vi "Fetch N - Blob.vi"(8 "error in (no error)":errorcluster, 9 "n rows (-1:all)":i32=-1, 11 "SQLite3LV Cursor in":refnum<class "cursor.lvclass">) -> (0 "error out":errorcluster, 1 "rows finished?":bool, 2 "result":string[][](array[string]), 3 "SQLite3LV Cursor out":refnum<class "cursor.lvclass">)   [LabVIEW 2014, in "SQLite3LV.lvlib" / "cursor.lvclass"]
uses:
  cursor.lvclass
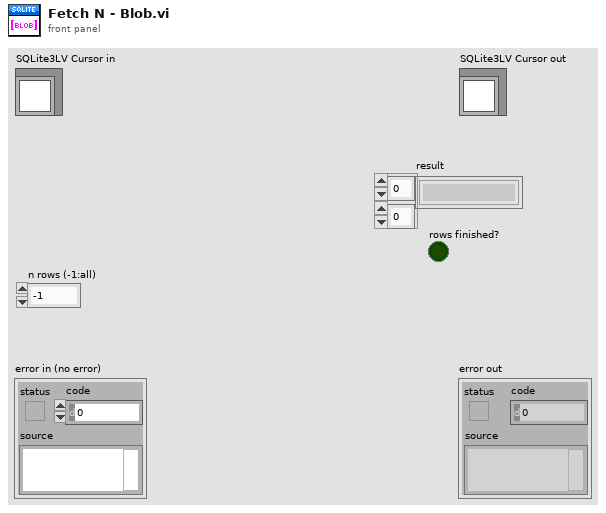
[diagram p1: front panel]
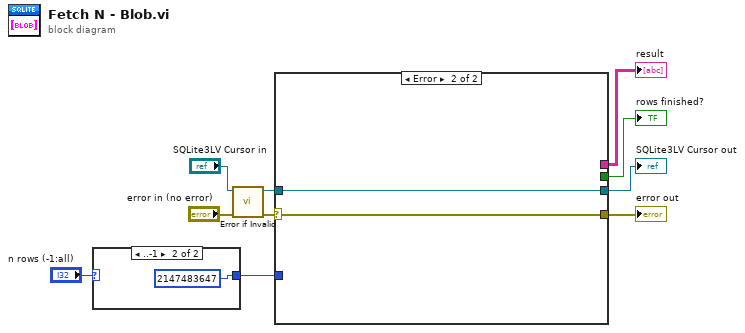
[diagram p0: block diagram]
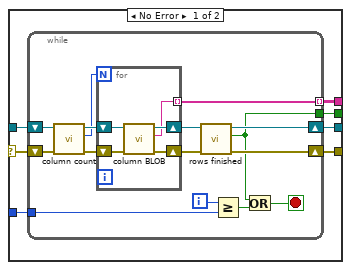
[diagram p3: hidden frame]
diagram:
  n1 = case shown="..-1" "n rows (-1:all)" {
    selector: "n rows (-1:all)" -> [w11 _]
    tunnel: [w11 2147483647 ("n rows (-1:all)")] -> w7
    frame Default {
    }
    frame ..-1 {
    }
  }
  n2 = call "Error if Invalid.vi"("error in (no error)"="error in (no error)", "SQLite3LV Cursor in"="SQLite3LV Cursor in") -> ("error out"=w2:errorcluster, "SQLite3LV Cursor out"=w3:refnum<class "cursor.lvclass">)  [unwired: 8 in]
  n3 = case shown="Error" w2 {
    selector: w2 -> [w18 w41]
    tunnel: [w15 w41] -> w10
    tunnel: [w17 w40] -> w9
    tunnel: w3 -> [w19 w40]
    tunnel: w7 -> [w14 _]
    tunnel: [w16 _] -> w6
    tunnel: [w13 _] -> w1
    frame No Error {
      n4 = while {
        shift-right: [w32] -> w17
        shift-left: w19 -> [w34]
        shift-right: [w27] -> w15
        shift-left: w18 -> [w30]
        tunnel: [w26] -> w16 mode=indexing
        tunnel: w14 -> [w24]
        tunnel: [w21] -> w13
        i -> [w25]
        stop <- w23 stop-if-true
        n5 = call "column count.vi"("error in (no error)"=w30, "SQLite3LV Cursor in"=w34) -> ("error out"=w29:errorcluster, "# of columns"=w20:i32, "SQLite3LV Cursor out"=w33:refnum<class "cursor.lvclass">)  [unwired: 7 in]
        n6 = for {
          N: w20 -> [_]
          shift-right: [w38] -> w31
          shift-left: w33 -> [w39]
          tunnel: [w37] -> w26 mode=indexing
          shift-right: [w35] -> w28
          shift-left: w29 -> [w36]
          n7 = call "column BLOB.vi"("error in (no error)"=w36, "SQLite3LV Cursor in"=w39) -> ("error out"=w35:errorcluster, "BLOB"=w37:string, "SQLite3LV Cursor out"=w38:refnum<class "cursor.lvclass">)  [unwired: 7 in]
        }
        n8 = call "rows finished"("error in (no error)"=w28, "SQLite3LV Cursor in"=w31) -> ("error out"=w27:errorcluster, "rows finished?"=w21:bool, "SQLite3LV Cursor out"=w32:refnum<class "cursor.lvclass">)  [unwired: 7 in]
        n9 = Greater Or Equal?(x=w25, y=w24) -> (x >= y?=w22:bool)
        n10 = Or(x=w21, y=w22) -> (x .or. y?=w23:bool)
      }
    }
    frame Error {
    }
  }
  "error out" <- w10
  "SQLite3LV Cursor out" <- w9
  "result" <- w6
  "rows finished?" <- w1
